vi "Actor Core.vi"(8 "error in":errorcluster, 11 "Nested in":refnum<class "MainController.lvclass">) -> (0 "error out":errorcluster, 3 "Actor out":refnum<class "Actor.lvclass">)   [LabVIEW 2020, in "MainController.lvlib" / "MainController.lvclass"]
doc: "(<B>Filename</B>: Actor Framework.lvlib:Actor.lvclass:Actor Core.vi)\n\nReceives messages to the actor, reacts to them, and initiates any error handling that may shut the actor down.\n\nDescendant classes may override this VI to append parallel tasks for the actor to complete while it handles messages. Overrides use the Call Parent Method node."
uses:
  MainController.lvclass
  C:/Program Files (x86)/National Instruments/LabVIEW 2020/vi.lib/ActorFramework/Actor/Actor.lvclass
  <vilib>/ActorFramework/Actor/Actor.lvclass
  MainController.lvclass/MainController.ctl
  <vilib>/ActorFramework/Actor/Actor.lvclass/Actor.ctl
  <vilib>/ActorFramework/Message Enqueuer/Message Enqueuer.lvclass/Message Enqueuer.ctl
  Write Main Pane.vi
  Write AppBar SubPanel.vi
  Write AppBar Splitter.vi
  Write Charm SubPanel.vi
  Write Charm Splitter.vi
  Write Title.vi
  Write UI VI Ref.vi
  <vilib>/ActorFramework/Message Enqueuer/Init from Existing Queue.vi
  <vilib>/ActorFramework/Message Enqueuer/Enqueue.vi
  <vilib>/ActorFramework/Stop Msg/Stop Msg.lvclass
  C:/Program Files (x86)/National Instruments/LabVIEW 2020/vi.lib/ActorFramework/Message/Message.lvclass
  <vilib>/ActorFramework/Message Priority Queue/Priority Enqueue.vi
  <vilib>/ActorFramework/Message Enqueuer/Message Enqueuer.lvclass
panel:
  out "Title":string="Title"
  out "Time":string
  out "Date":string
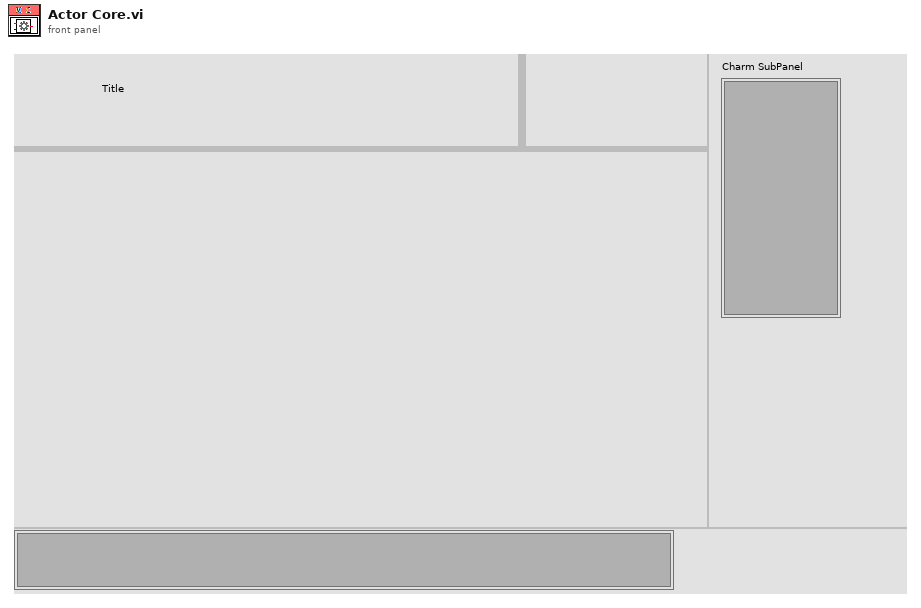
[diagram p1: front panel]
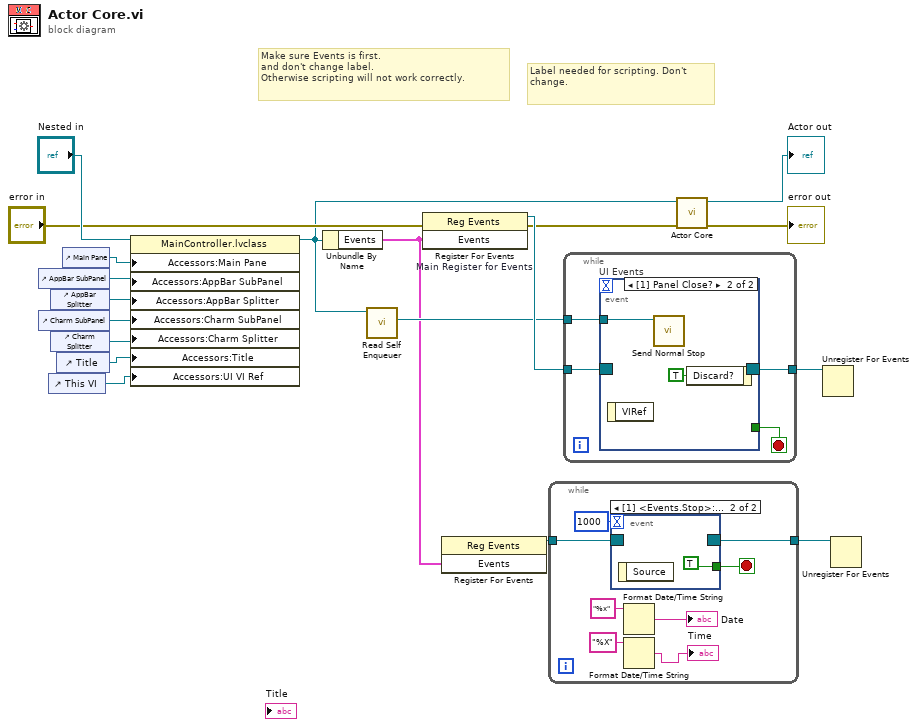
[diagram p0: block diagram]
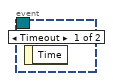
[diagram p2: hidden frame]
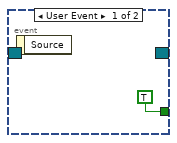
[diagram p3: hidden frame]
diagram:
  # "Label needed for scripting. Don't change."
  # "Make sure Events is first.\nand don't change label.\nOtherwise scripting will not work correctly."
  n1 = control-ref of="AppBar SubPanel"() -> (w6:refnum<vi>)
  n2 = control-ref of="Charm SubPanel"() -> (w4:refnum<vi>)
  n3 = control-ref of="This VI"() -> (w1:refnum<vi>)
  n4 = control-ref of="AppBar Splitter"() -> (w5:refnum<vi>)
  n5 = control-ref of="Charm Splitter"() -> (w3:refnum<vi>)
  n6 = control-ref of="Title"() -> (w2:refnum<vi>)
  n7 = control-ref of="Main Pane"() -> (w7:refnum<vi>)
  n8 = property class="MainController.lvclass"(reference="Nested in", "Accessors:Main Pane"=w7, "Accessors:AppBar SubPanel"=w6, "Accessors:AppBar Splitter"=w5, "Accessors:Charm SubPanel"=w4, "Accessors:Charm Splitter"=w3, "Accessors:Title"=w2, "Accessors:UI VI Ref"=w1) -> (reference out=w8:refnum<class "MainController.lvclass">)  [unwired: 1 in, 1 out]
  n9 = Unbundle By Name(w8) -> ("Events"=w11:cluster{"Stop":refnum<user-event>})
  n10 = call <vilib>:"Read Self Enqueuer.vi"("Actor"=w8) -> ("Self Enqueuer"=w14:refnum<class "Message Enqueuer.lvclass">)  [unwired: 10 in]
  n11 = register-events "Main Register for Events"(error in="error in", w11) -> (reference out=w17:refnum<event-registration>, error out=w12:errorcluster)  [unwired: 1 in]
  n12 = register-events ("Main Register for Events")(w11) -> (reference out=w10:refnum<event-registration>)  [unwired: 2 in, 1 out]
  n13 = while {
    tunnel: w10 -> [w26]
    tunnel: [w20] -> w9
    stop <- w25 stop-if-true
    n14 = event shown="[1] <Events.Stop>: User Event" {
      selector: w26 -> [_ _]
      dyn-events: [_ _] -> w20
      timeout: 1000 -> [_ _]
      tunnel: [_ TRUE] -> w25
      event Timeout {
        n15 = event-data() -> ()  [unwired: 1 in, 1 out]
      }
      event User Event {
        n16 = event-data() -> ()  [unwired: 1 in, 1 out]
      }
    }
    n17 = Format Date/Time String(time format string (%c)="%x") -> (date/time string=→"Date":string)  [unwired: 2 in]
    n18 = Format Date/Time String(time format string (%c)="%X") -> (date/time string=→"Time":string)  [unwired: 2 in]
  }
  n19 = while {
    tunnel: w17 -> [w32]
    tunnel: [w30] -> w16
    tunnel: w14 -> [w29]
    stop <- w31 stop-if-true
    n20 = event "UI Events" shown="[1] Panel Close?" {
      selector: w32 -> [_ _]
      dyn-events: [_ _] -> w30
      timeout: _ -> [_ _]
      tunnel: [TRUE _] -> w31
      tunnel: w29 -> [_ w34]
      event User Event {
        n21 = event-data() -> ()  [unwired: 1 in, 1 out]
      }
      event Panel Close? {
        n22 = event-data() -> ()  [unwired: 1 in, 1 out]
        n23 = call <vilib>:"Send Normal Stop.vi"("Message Enqueuer"=w34) -> ()  [unwired: 10 in, 1 out]
        n24 = event-data("Discard?"=TRUE) -> ()  [unwired: 1 in, 1 out]
      }
    }
  }
  n25 = call-parent "Actor Core.vi"("error in"=w12, "Actor in"=w8) -> ("error out"=→"error out":errorcluster, "Actor out"=→"Actor out":refnum<class "Actor.lvclass">)  [unwired: 8 in]
  n26 = Unregister For Events(event registration refnum=w16) -> ()  [unwired: 1 in, 1 out]
  n27 = Unregister For Events(event registration refnum=w9) -> ()  [unwired: 1 in, 1 out]
